vi "DP-Coerce Sampling Rate.vi"(0 "StimGen (out) in":T1, 11 "error in (no error)":errorcluster) -> (4 "StimGen (out) out":T1, 15 "error out":errorcluster)   [LabVIEW 2020]
uses:
  Typedefs/DP-StimGen.ctl
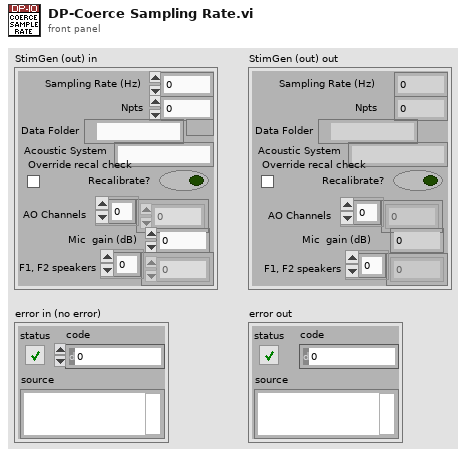
[diagram p1: front panel]
types:
  T1 = typedef "DP-StimGen.ctl" = cluster{"Sampling Rate (Hz)":dbl, "Npts":i32, "Data Folder":path, "Acoustic System":string, "Recalibrate?":bool, "AO Channels":i32[], "Mic  gain (dB)":dbl, "F1, F2 speakers":i32[], "Override recal check":bool}
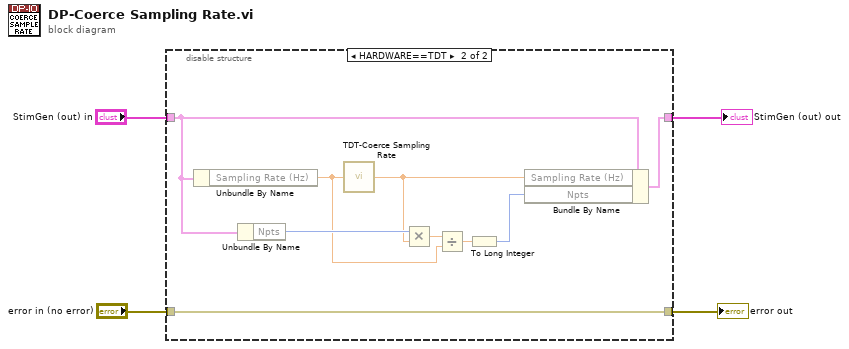
[diagram p0: block diagram]
diagram:
  n1 = disable-structure shown="HARDWARE==TDT" {
    disable-tunnel: "StimGen (out) in" -> [w6 w13]
    disable-tunnel: [w6 w15] -> w3
    disable-tunnel: [w5 w14] -> w2
    disable-tunnel: "error in (no error)" -> [w5 w14]
    frame condition #0 (active) {
    }
    frame condition #1 {
      n2 = Unbundle By Name(w13) -> ("Sampling Rate (Hz)"=w9:dbl)
      n3 = Unbundle By Name(w13) -> ("Npts"=w12:i32)
      n4 = call "TDT-Coerce Sampling Rate.vi"("Fs (Hz)"=w9) -> ("Coerced"=w11:dbl)
      n5 = Multiply(x=w12, y=w11) -> (x*y=w10:dbl)
      n6 = Divide(x=w10, y=w9) -> (x/y=w8:dbl)
      n7 = To Long Integer(number=w8) -> (32bit integer=w7:i32)
      n8 = Bundle By Name(cluster=w13, "Sampling Rate (Hz)"=w11, "Npts"=w7) -> (w15:T1)
    }
  }
  "StimGen (out) out" <- w3
  "error out" <- w2
